vi "Reduce Samples.vi"() -> ()   [LabVIEW 2016]
panel:
  out "Table":string[][](table)
  in  "stop":bool
  out "Sine":dynamicdata(graph)
  in  "Enable":bool=TRUE
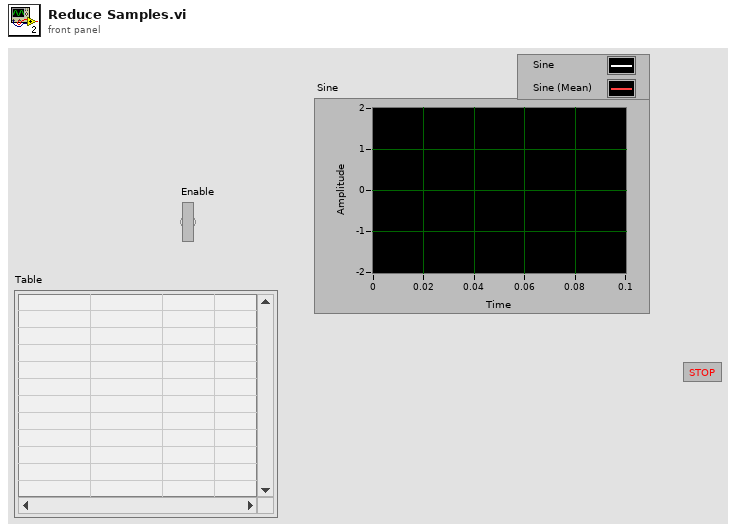
[diagram p1: front panel]
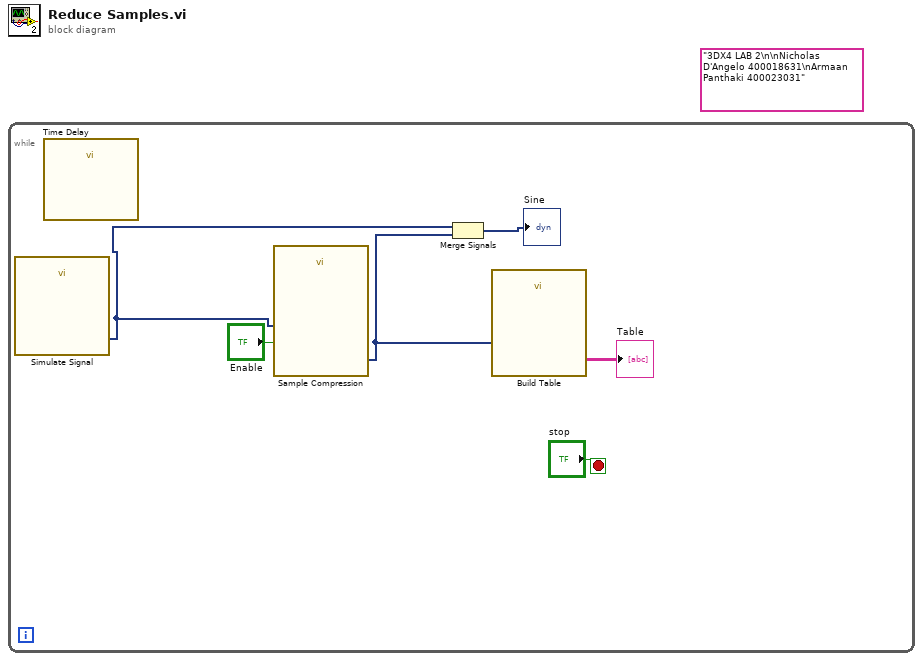
[diagram p0: block diagram]
diagram:
  (unwired) "3DX4 LAB 2\n\nNicholas D'Angelo 400018631\nArmaan Panthaki 400023031"
  n1 = while {
    stop <- "stop" stop-if-true
    n2 = call "Simulate Signal"() -> ("Sine"=w5:dynamicdata)  [unwired: 14 in, 1 out]
    n3 = call "Time Delay"() -> ()  [unwired: 11 in, 1 out]
    n4 = call "Sample Compression"("Enable"="Enable", "Signals"=w5) -> ("Mean"=w1:dynamicdata)  [unwired: 7 in, 2 out]
    n5 = Merge Signals(w5, w1) -> (→"Sine":dynamicdata)
    n6 = call "Build Table"("Signals"=w1) -> ("Table"=→"Table":string[][])  [unwired: 4 in, 6 out]
  }
